vi "Lab.07_EMG.vi"() -> ()   [LabVIEW 2016]
uses:
  <vilib>/Analysis/2dsp.llb/Real FFT.vi
  <vilib>/Analysis/baseanly.llb/Mean (DBL).vi
  <vilib>/measure/maspectr.llb/FFT Power Spectrum and PSD for N Chan.vi
  <vilib>/measure/NI_MAPro.lvlib
  <vilib>/Analysis/NI_AALPro.lvlib
  <vilib>/Analysis/NI_AALBase.lvlib
panel:
  out "amplitude":dbl
  out "LED out":bool
  out "EMG signal":dynamicdata(graph)
  out "relax/contract":bool
  out "instruction":string
  out "frequency":cluster{"f0":dbl, "df":dbl, "magnitude":dbl[]}[](graph)
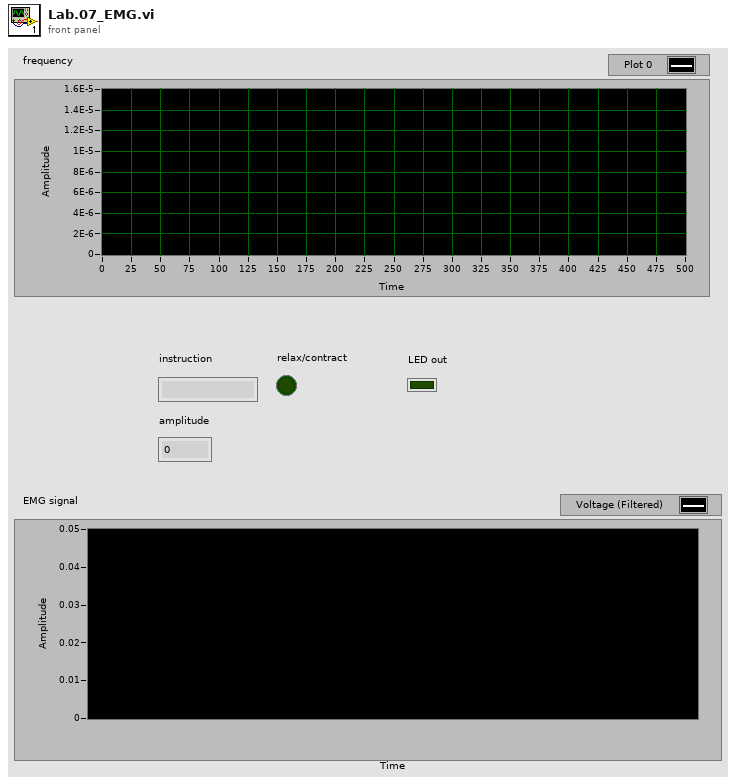
[diagram p1: front panel]
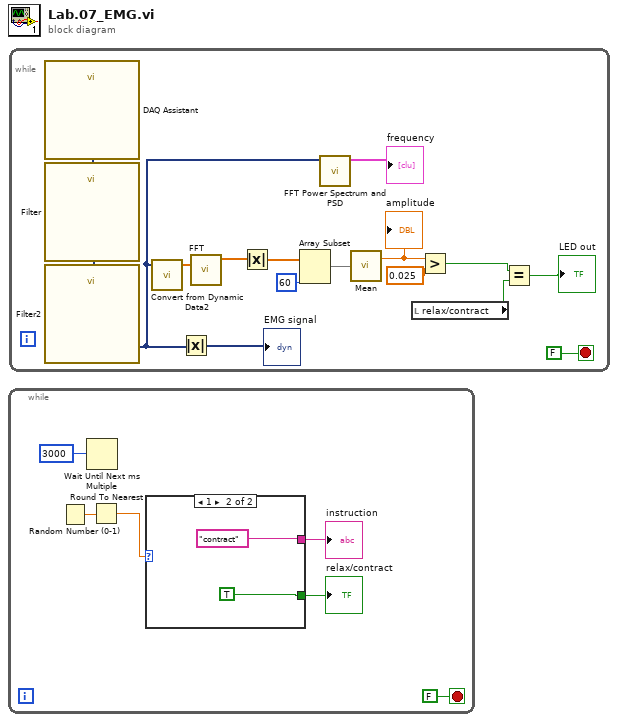
[diagram p0: block diagram]
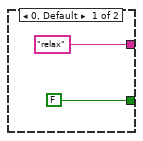
[diagram p2: hidden frame]
diagram:
  n1 = while {
    stop <- FALSE stop-if-true
    n2 = Random Number (0-1)() -> (number: 0 to 1=w4:dbl)
    n3 = Wait Until Next ms Multiple(millisecond multiple=3000) -> ()  [unwired: 1 out]
    n4 = Round To Nearest(number=w4) -> (nearest integer value=w3:dbl)
    n5 = case shown="1" w3 {
      tunnel: ["relax" "contract"] -> w2
      tunnel: [FALSE TRUE] -> w1
      frame 0, Default {
      }
      frame 1 {
      }
    }
    "instruction" <- w2
    "relax/contract" <- w1
  }
  n6 = while {
    stop <- FALSE stop-if-true
    n7 = call "DAQ Assistant"() -> ("data"=w26:dynamicdata)  [unwired: 16 in, 3 out]
    n8 = call "Filter"("Signal"=w26) -> ("Filtered Signal"=w14:dynamicdata)  [unwired: 9 in, 1 out]
    n9 = call "Filter2"("Signal"=w14) -> ("Filtered Signal"=w13:dynamicdata)  [unwired: 9 in, 1 out]
    n10 = call "Convert from Dynamic Data2"("Dynamic Data Type"=w13) -> ("Array"=w12:dbl[])  [unwired: 3 in]
    n11 = Absolute Value(x=w13) -> (abs(x)=→"EMG signal":dynamicdata)
    n12 = call-poly <vilib>:"FFT.vi"("X"=w12) -> ("FFT {X}"=w22:cdb[])  [unwired: 9 in, 1 out]
    n13 = Absolute Value(x=w22) -> (abs(x)=w21:dbl[])
    n14 = Array Subset(array=w21, length=60) -> (w19:dbl[])  [unwired: 1 in]
    n15 = call-poly <vilib>:"FFT Power Spectrum and PSD.vi"("time signals"=w13) -> ("Power Spectrum / PSD"=→"frequency":cluster{"f0":dbl, "df":dbl, "magnitude":dbl[]}[])  [unwired: 7 in, 3 out]
    n16 = call-poly <vilib>:"Mean.vi"("X"=w19) -> ("mean"=w11:dbl)  [unwired: 1 out]
    "amplitude" <- w11
    n17 = local read "relax/contract"() -> (w16:bool)
    n18 = Greater?(x=w11, y=0.025) -> (0:w17:bool)
    n19 = Equal?(x=w17, y=w16) -> (x = y?=→"LED out":bool)
  }
